vi "LoginDialogBox.vi"(10 "AppKey":string, 11 "URL":string caption="Base URL") -> (1 "URL out":string caption="URL", 2 "AppKey out":string caption="API Key", 3 "OK?":bool caption="OK")   [LabVIEW 2016]
panel:
  in  "Help":bool caption="Cancel"
  in  "Cancel":bool
  in  "OK":bool caption="OK2"
  # "Please enter your SystemLink credentials"
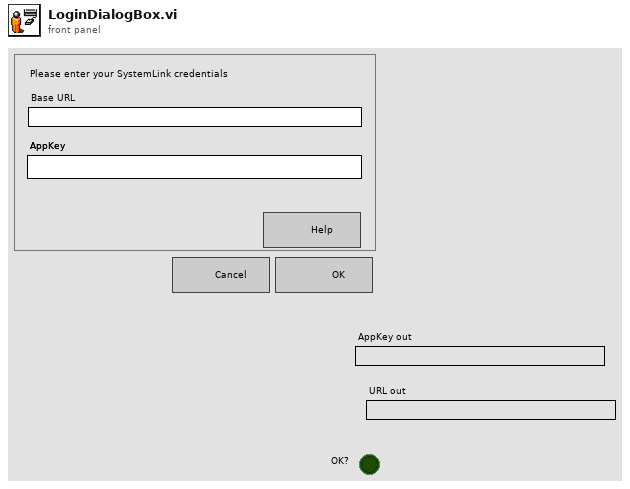
[diagram p1: front panel]
types:
  T1 = enum8{"Enabled", "Disabled", "Disabled and Grayed Out"}
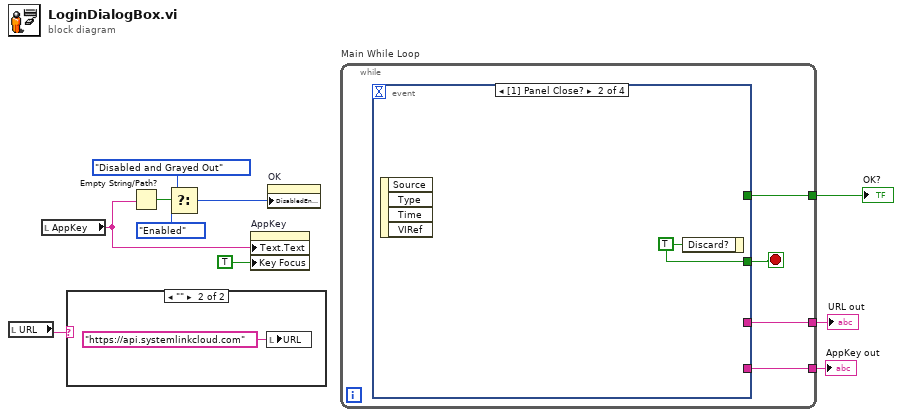
[diagram p0: block diagram]
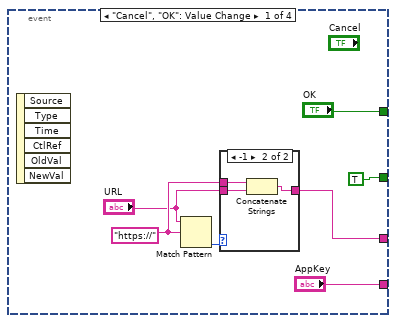
[diagram p3: hidden frame]
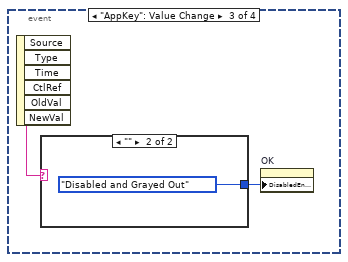
[diagram p5: hidden frame]
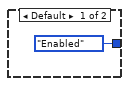
[diagram p6: hidden frame]
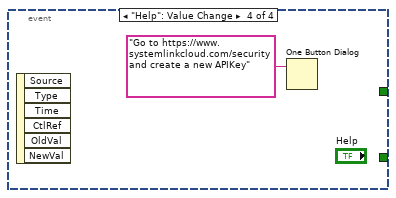
[diagram p7: hidden frame]
diagram:
  n1 = local read "URL"() -> (w9:string)
  n2 = local read "AppKey"() -> (w5:string)
  n3 = case shown="\"\"" w9 {
    frame Default {
    }
    frame "" {
      n4 = local write "URL"("https://api.systemlinkcloud.com" ("URL")) -> ()
    }
  }
  n5 = Empty String/Path?(string/path=w5) -> (empty?=w4:bool)
  n6 = Select(t=T1."Disabled and Grayed Out" ("Disabled"), s=w4, f=T1."Enabled" ("Disabled")) -> (s? t:f=w1:T1)
  n7 = property on="AppKey" class="Str"("Text.Text"=w5, "Key Focus"=TRUE ("focus on")) -> ()  [unwired: 2 in, 2 out]
  n8 = property on="OK" class="Bool"("DisabledEnum"=w1) -> ()  [unwired: 2 in, 2 out]
  n9 = while "Main While Loop" {
    tunnel: [w14] -> w8
    tunnel: [w13] -> w7
    tunnel: [w12] -> w6
    stop <- w15 stop-if-true
    n10 = event shown="[1] Panel Close?" {
      selector: _ -> [_ _ _ _]
      dyn-events: _ -> [_ _ _ _]
      timeout: _ -> [_ _ _ _]
      tunnel: [TRUE w27 _ _] -> w15
      tunnel: ["OK" _ _ _] -> w14
      tunnel: [w16 _ _ _] -> w13
      tunnel: ["AppKey" _ _ _] -> w12
      event "Cancel", "OK": Value Change {
        w18 = "https://" ("URL")
        n11 = event-data() -> ()  [unwired: 1 in, 6 out]
        n12 = Match Pattern(string="URL", regular expression=w18) -> (offset past match=w19:i32)  [unwired: 1 in, 3 out]
        n13 = case shown="-1" w19 {
          tunnel: w18 -> [_ w26]
          tunnel: "URL" -> [w23 w25]
          tunnel: [w23 w24] -> w16
          frame Default {
          }
          frame -1 {
            n14 = Concatenate Strings(w26, w25) -> (w24:string)
          }
        }
      }
      event Panel Close? {
        w27 = TRUE ("Discard?")
        n15 = event-data() -> ()  [unwired: 1 in, 4 out]
        n16 = event-data("Discard?"=w27) -> ()  [unwired: 1 in, 1 out]
      }
      event "AppKey": Value Change {
        n17 = event-data() -> ("NewVal"=w28:string)  [unwired: 1 in, 5 out]
        n18 = case shown="\"\"" w28 {
          tunnel: [T1."Enabled" ("Disabled") T1."Disabled and Grayed Out" ("Disabled")] -> w29
          frame Default {
          }
          frame "" {
          }
        }
        n19 = property on="OK" class="Bool"("DisabledEnum"=w29) -> ()  [unwired: 2 in, 2 out]
      }
      event "Help": Value Change {
        n20 = event-data() -> ()  [unwired: 1 in, 6 out]
        n21 = One Button Dialog(message="Go to https://www.systemlinkcloud.com/security and create a new APIKey") -> ()  [unwired: 1 in, 1 out]
      }
    }
  }
  "AppKey out" <- w6
  "URL out" <- w7
  "OK?" <- w8
